vi "Rio_Shutdown (DONE).vi"(8 "error in (no error)":errorcluster) -> (0 "error out":errorcluster)   [LabVIEW 2017]
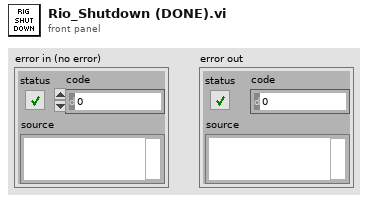
[diagram p1: front panel]
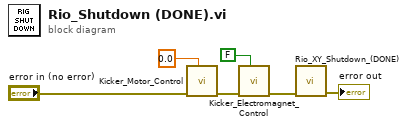
[diagram p0: block diagram]
diagram:
  n1 = call "Kicker_Motor_Control.vi"("Duty Cycle"=0.0, "error in"="error in (no error)") -> ("error out"=w1:errorcluster)  [unwired: 9 in]
  n2 = call "Kicker_Electromagnet_Control.vi"("Mag Enable"=FALSE, "error in"=w1) -> ("error out"=w5:errorcluster)  [unwired: 9 in]
  n3 = call "Rio_XY_Shutdown_(DONE).vi"("error in (no error)"=w5) -> ("error out"=→"error out":errorcluster)  [unwired: 10 in]
